vi "SaveMultipleArraysAsText.vi"() -> ()   [LabVIEW 2018, in "RW_Protocols.lvlib"]
uses:
  RW_Protocols.lvlib
panel:
  out "unsigned 16bit integer":u16[][](array[numeric])
  in  "Target Folder":path=path "D:/Data/Mai/test target"
  in  "HOL out":cdb[][](array[numeric])
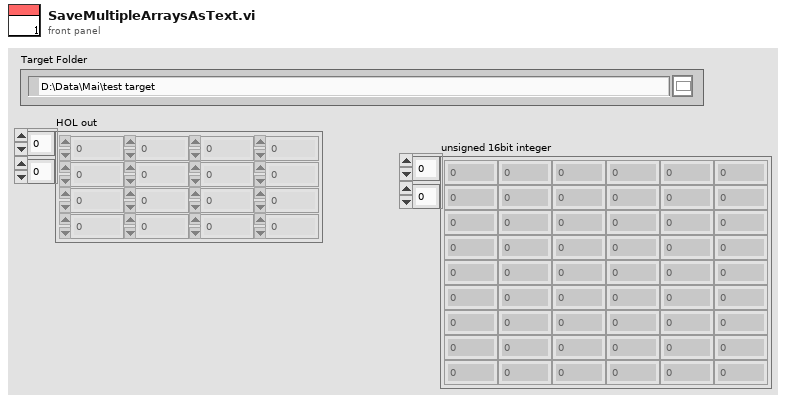
[diagram p1: front panel]
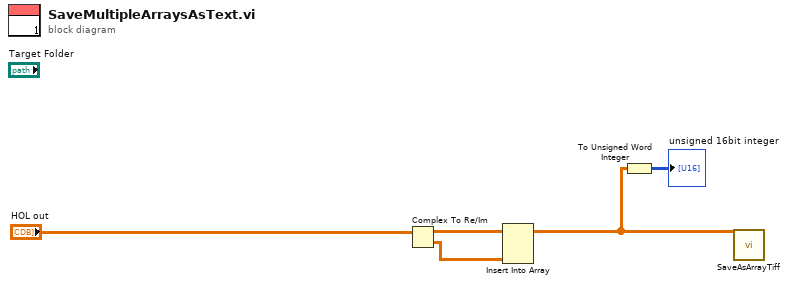
[diagram p0: block diagram]
diagram:
  n1 = Complex To Re/Im(x + iy="HOL out") -> (x=w4:dbl[][], y=w3:dbl[][])
  n2 = Insert Into Array(array=w4, new element=w3) -> (w2:dbl[][])  [unwired: 2 in]
  n3 = To Unsigned Word Integer(number=w2) -> (unsigned 16bit integer=→"unsigned 16bit integer":u16[][])
  n4 = call "SaveAsArrayTiff.vi"("u16 array"=w2) -> ()  [unwired: 11 in]
